vi "Class DVR API Generator.vi"(6 "DVR API Suffix":string=" API", 8 "error in (no error)":errorcluster, 9 "DVR API Folder Name":string="APIs", 10 "Method Folder Name":string="Methods", 11 "Class Path":path) -> (0 "error out":errorcluster)   [LabVIEW 2016, in "SLL Scripting.lvlib"]
doc: "Generates DVR based APIs for the class methods. \n\nSpecify the \n1. Class path, \n2. Methods folder where the class methods are present,\n3. DVR API folder where the DVR APIs needs to be created,\n4. Suffix for the DVR APIs to be generated"
uses:
  SLL Scripting.lvlib
  _Class DVR API Generator/SLL Class DVR API Generator.lvlib
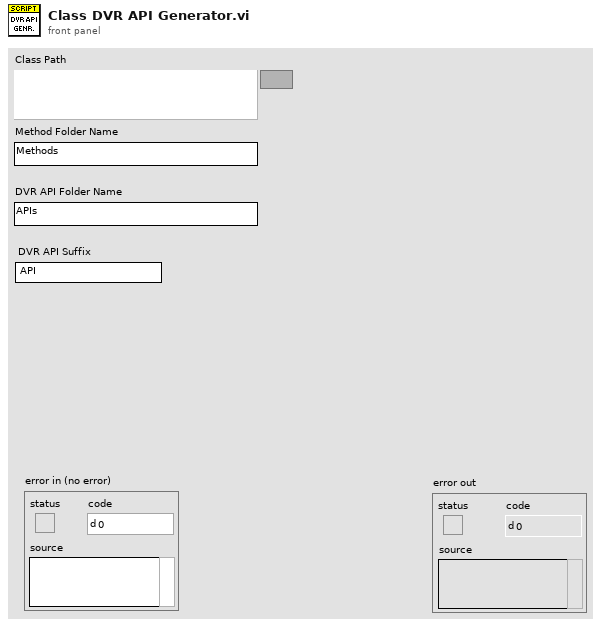
[diagram p1: front panel]
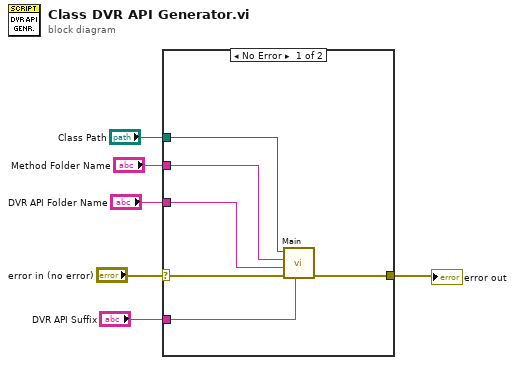
[diagram p0: block diagram]
diagram:
  n1 = case shown="No Error" "error in (no error)" {
    selector: "error in (no error)" -> [w12 w13]
    tunnel: [w11 w13] -> w5
    tunnel: "Class Path" -> [w10 _]
    tunnel: "Method Folder Name" -> [w9 _]
    tunnel: "DVR API Folder Name" -> [w8 _]
    tunnel: "DVR API Suffix" -> [w7 _]
    frame No Error {
      n2 = call "Main.vi"("DVR API Suffix"=w7, "error in (no error)"=w12, "DVR API Folder Name"=w8, "Method Folder Name"=w9, "Class Path"=w10) -> ("error out"=w11:errorcluster)  [unwired: 6 in]
    }
    frame Error {
    }
  }
  "error out" <- w5
